vi "模拟器自动控制程序（轨迹跟踪）.vi"() -> ()   [LabVIEW 2012]
uses:
  <vilib>/Utility/error.llb/DialogType.ctl
  <vilib>/Platform/TimedLoop/XDataNode/timing_clust.ctl
  <vilib>/Platform/TimedLoop/XDataNode/nitl_modes.ctl
  <vilib>/Platform/TimedLoop/XDataNode/wakeup.ctl
  <vilib>/Instr/_visa.llb/VISA Configure Serial Port (Instr).vi
  <vilib>/DAQmx/create/channels.llb/DAQmx Create Channel (DO-Digital Output).vi
  <vilib>/Analysis/Matrix/Numeric/Conversions/Array To Matrix - RA2.vi
  <vilib>/Utility/file.llb/Write To Spreadsheet File (DBL).vi
  <vilib>/Platform/TimedLoop/XDataNode/XDataNode.xnode
  <vilib>/Platform/TimedLoop/XDataNode/XDNodeRunTimeDep.lvlib
  <vilib>/Analysis/Matrix/NI_Matrix.lvlib
  <vilib>/vision/NI_Vision_Development_Module.lvlib
  <vilib>/Analysis/NI_AALBase.lvlib
panel:
  out "Truster4":bool
  out "Truster 8":bool
  out "Truster  3":bool
  out "Truster 7":bool
  out "Truster 5":bool
  out "Truster  2":bool
  out "Truster 6":bool
  out "Truster1":bool
  out "定位点信息":T1(array[cluster]) {"Aspect Ratio" format="%.2f"; "Orientation" format="%.2f"; "Area" format="%.2f"; "Object Center"."Y" format="%.2f"; "Object Center"."X" format="%.2f"}
  out "alpha":dbl
  out "计时参数":dbl
  in  "卫星模拟器":enum32{"初始化", "运行监测"}(tab)
  out "读取缓冲区":string
  out "电流校正模式":bool
  out "软件使能":bool caption="软件使能(启动/停止)"
  out "电流校正中":bool caption="电流校正完成"
  out "E2PROM初始化结果":bool
  out "E2初始化完成":bool
  out "CRC校验和错误":bool
  out "串口通信错误":bool caption="串口通信故障"
  out "发送指令":string
  out "控制命令":string
  out "电机已启动":bool
  in  "采样率":i64=10
  in  "限制转速":dbl=500.0
  in  "ID号":u8=255 step=1 format="%#.0f"
  in  "最高转速":dbl=500.0
  in  "PWM周期":dbl=1599.0
  in  "最大力矩":dbl=2047.0
  in  "stop bits (10: 1 bit)":u16(ring)=10 caption="停止位" items=["1.0"=10, "1.5"=15, "2.0"=20]
  out "串口状态":bool
  in  "端口选择":refnum<visa-resource-name>="COM1"
  in  "波特率":u16(ring)=10 items=["   300", "   600", "   1200", "   2400", "   4800   ", "   9600", "   19200", "   38400", "   43000", "   56000", "   57600", "   115200"]
  in  "校验":enum16{"None", "Odd", "Even"}(ring)=enum."Even"
  in  "数据位":u16=8
  in  "打开":bool caption="stop"
  out "轨控信号":dbl
  in  "姿轨控开始":bool
  out "转速模式":bool
  out "转矩模式":bool
  out "故障":bool
  out "启停状态":bool
  in  "存储波形":bool
  in  "显示波形 停止显示":bool
  in  "开始记录":bool
  out "动量轮转矩":dbl format="%#_6f"
  out "动量轮转速":dbl format="%#_4f"
  out "X速率(cm/s)":dbl
  out "Y速率(cm/s)":dbl
  out "Y偏移量 (cm)":dbl
  out "X偏移量 (cm)":dbl
  out "相对偏角(deg)":dbl
  out "角速度(deg/s)":dbl
  out "设备ID":u8=255
  in  "模式选择":u16(ring)=1 items=["电流校正模式", "转矩模式", "转速模式", "开环测试模式"]
  in  "模式选择":bool
  in  "写指令字":dbl
  in  "清除故障":bool
  in  "停止电机":bool
  in  "启动电机":bool
  out "波形图":cluster{"转矩反馈":dbl, "转速反馈":dbl}(graph)
  in  "退出程序":bool caption="停止电机 2"
  in  "Floating":bool
  in  "缩放比例 (像素/cm)":dbl=4.099468
  in  "X中心校正":dbl
  in  "Y中心校正":dbl
  out "指令Y":dbl
  out "指令X":dbl
  out "指令角度":dbl
  out "alpha (deg)":dbl
  out "x >= y?":bool
  out "数值":dbl
  out "输出数组 6":dbl[](array[numeric])
  out "输出数组 7":dbl[](array[numeric])
  out "输出数组 10":dbl[](array[numeric])
  out "无符号字节数组 2":u8[](array[numeric])
  # "状态"
  # "设置"
  # "控制信号"
  # "参数确定"
  # "状态显示"
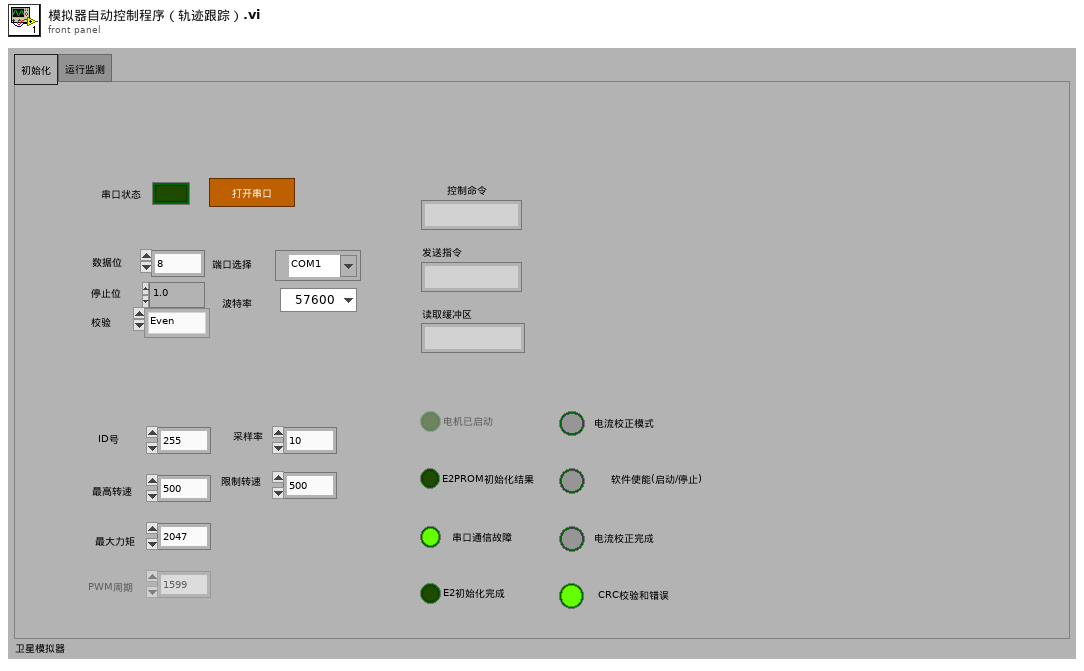
[diagram p1: front panel]
types:
  T1 = cluster{"Object Center":cluster{"X":sgl, "Y":sgl}, "Bounding Box":cluster{"X Left":i32, "Y Top":i32, "X Right":i32, "Y Bottom":i32}, "Area":sgl, "Orientation":sgl, "Aspect Ratio":sgl, "Nb Holes":i32}[]
  T2 = typedef "XDNodeRunTimeDep.lvlib/timing_clust.ctl" = cluster{"Expected End [f-1]":u64, "Actual End [f-1]":u64, "Finished Late? [f-1]":bool, "Expected End [i-1]":u64, "Actual End [i-1]":u64, "Finished Late? [i-1]":bool, "Expected Start [i]":u64, "Actual Start [i]":u64, "Expected Start [f]":u64, "Actual Start [f]":u64, "Source Name":string, "Structure Name":string, "Period":i64, "Deadline":i64, "Offset":i64, "Start":i64, "Priority":i32, "Timeout":i32, "Mode":T3, "Wakeup Reason":T4, "Error":errorcluster, "Source Type":string, "Secondary Source Type":string, "Global End Time":u64, "Global Start Time":u64, "Frame Duration":u64, "Iteration Duration":u64, "Assigned CPU":i32, "I/O Scan Engine Mode":u32}
  T3 = typedef "XDNodeRunTimeDep.lvlib/nitl_modes.ctl" = enum32{"No Change", "Process missed periods, maintain original phase", "Discard missed periods, maintain original phase", "Process missed periods, ignore original phase", "Discard missed periods, ignore original phase"}
  T4 = typedef "XDNodeRunTimeDep.lvlib/wakeup.ctl" = enum32{"Normal", "Aborted", "Asynchronous wakeup", "Timing source error", "Timed loop error", "Timeout"}
  T5 = cluster{"Objects":u16, "Threshold":i32, "Reject Border":bool, "Fill Holes":bool, "Min Object Size":bool, "Min Size":i32, "Max Object Size":bool, "Max Size":i32, "Show Search Area":bool, "Show Center":bool, "Show Bounding Box":bool}
  T6 = typedef "DialogType.ctl" = u16
  T7 = typedef "NI_Matrix.lvlib/RealMatrix.ctl" = dbl[][]
  T8 = typedef "IMAQ Image.ctl" = refnum<image>
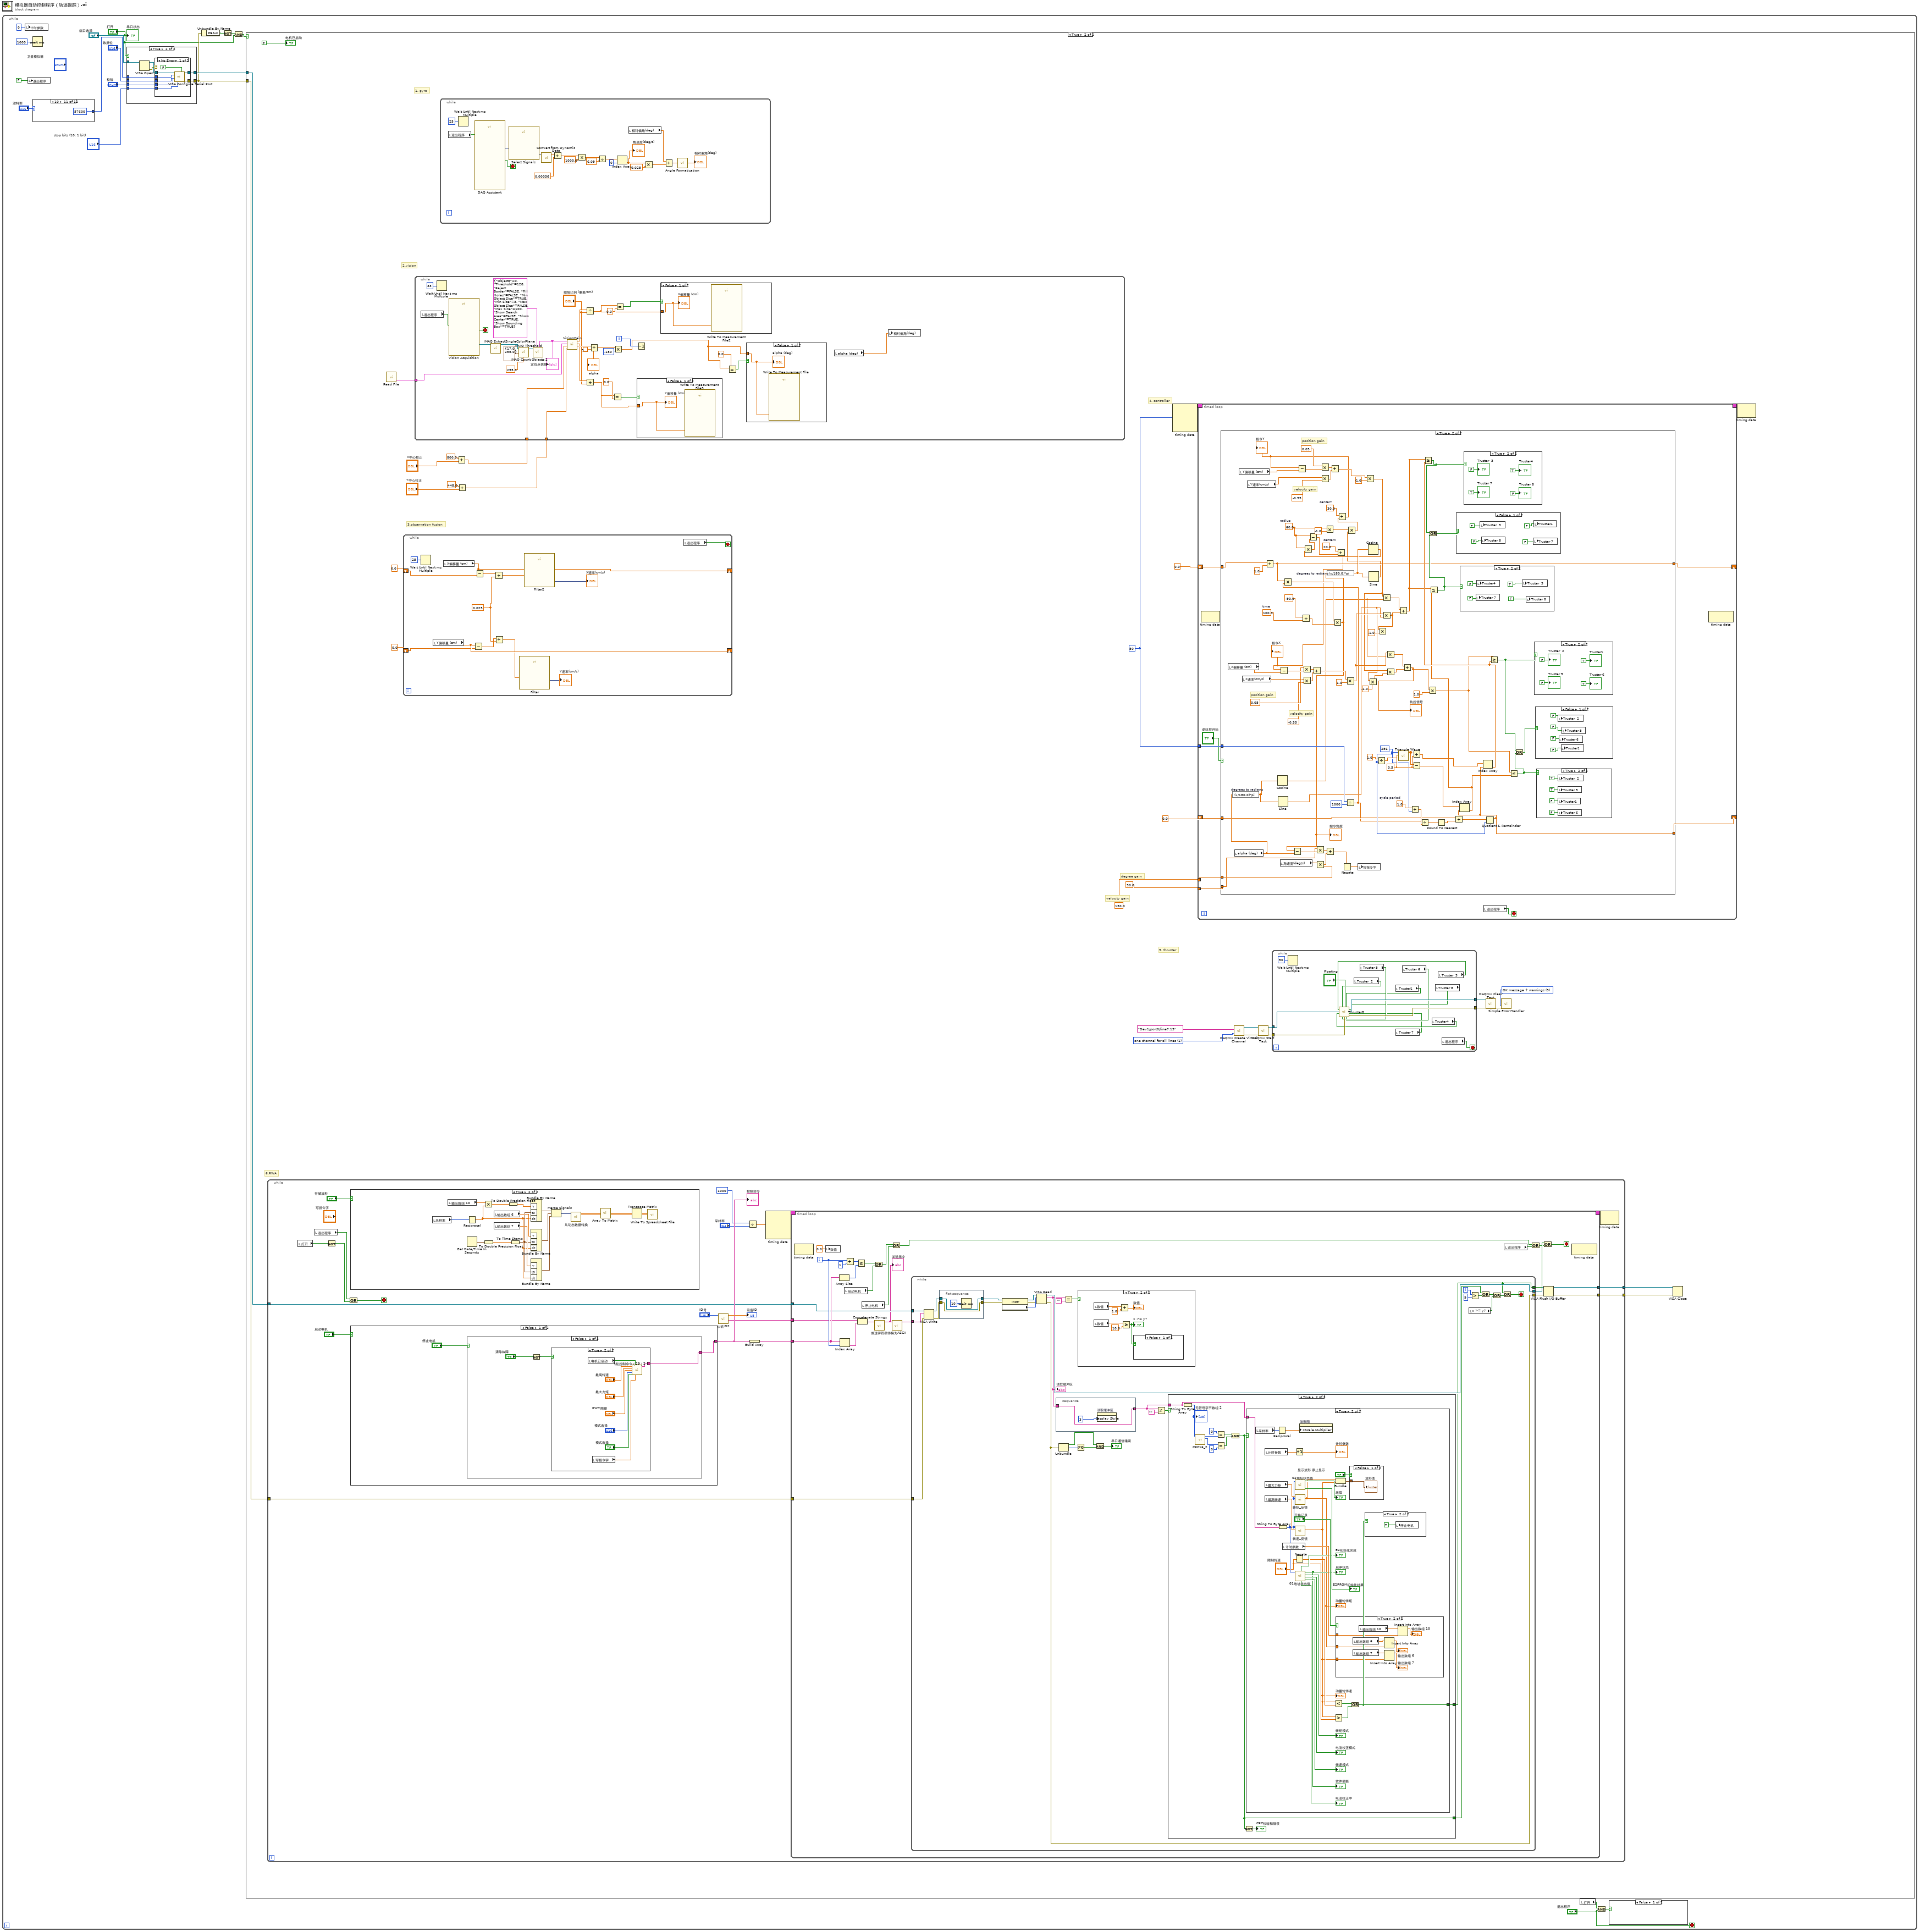
[diagram p0: block diagram]
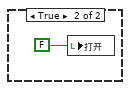
[diagram p2: hidden frame]
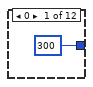
[diagram p5: hidden frame]
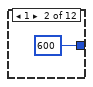
[diagram p6: hidden frame]
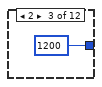
[diagram p7: hidden frame]
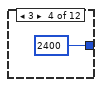
[diagram p8: hidden frame]
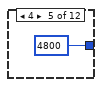
[diagram p9: hidden frame]
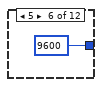
[diagram p10: hidden frame]
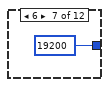
[diagram p11: hidden frame]
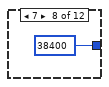
[diagram p12: hidden frame]
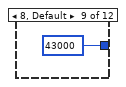
[diagram p13: hidden frame]
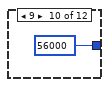
[diagram p14: hidden frame]
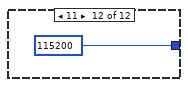
[diagram p15: hidden frame]
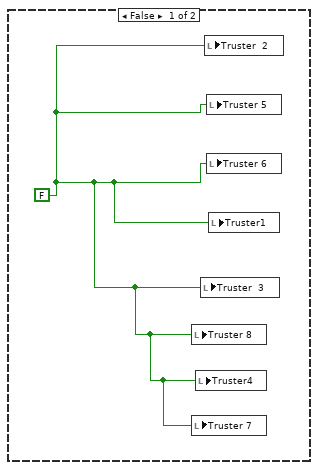
[diagram p17: hidden frame]
diagram:
  n1 = while {
    stop <- "退出程序" stop-if-true
    n2 = local write "计时参数"(0) -> ()
    n3 = local write "退出程序"(FALSE ("退出程序")) -> ()
    n4 = Wait (ms)(milliseconds to wait=u32 1000 ("等待时间（毫秒）")) -> ()  [unwired: 1 out]
    n5 = case shown="10" "波特率" {
      tunnel: [300 600 1200 2400 4800 9600 19200 38400 43000 56000 57600 115200] -> w17
      frame 0 {
      }
      frame 1 {
      }
      frame 2 {
      }
      frame 3 {
      }
      frame 4 {
      }
      frame 5 {
      }
      frame 6 {
      }
      frame 7 {
      }
      frame 8, Default {
      }
      frame 9 {
      }
      frame 10 {
      }
      frame 11 {
      }
    }
    n6 = case shown="True" "打开" {
      tunnel: w17 -> [_ w28]
      tunnel: "数据位" -> [_ w27]
      tunnel: "校验" -> [_ w26]
      tunnel: "端口选择" -> [_ w25]
      tunnel: [_ w22] -> w7
      tunnel: [_ w21] -> w6
      tunnel: "stop bits (10: 1 bit)" -> [_ w20]
      frame False {
      }
      frame True {
        n7 = VISA Open(VISA resource name=w25) -> (VISA resource name=w24:refnum<visa-resource-name>, error out=w23:errorcluster)  [unwired: 1 in, 3 out]
        n8 = case shown="No Error" w23 {
          tunnel: w28 -> [w36 _]
          tunnel: w27 -> [w35 _]
          tunnel: w26 -> [w34 _]
          tunnel: w24 -> [w33 _]
          tunnel: [w32 _] -> w22
          tunnel: [w31 _] -> w21
          tunnel: w20 -> [w30 _]
          frame No Error {
            n9 = call-poly "VISA Configure Serial Port"("VISA resource name"=w33, "Enable Termination\nChar (T)"=FALSE ("Enable Termination\nChar (T)"), "baud rate (9600)"=w36, "data bits (8)"=w35, "parity (0:none)"=w34, "stop bits (10: 1 bit)"=w30) -> ("VISA resource name out"=w32:refnum<visa-resource-name>, "error out"=w31:errorcluster)  [unwired: 2 in, 6 out]
          }
          frame Error {
          }
        }
      }
    }
    n10 = Unbundle By Name(w6) -> ("status"=w12:bool)
    n11 = Not(x=w12) -> (.not. x?=w11:bool)
    n12 = And(x=w11, y="打开") -> (x .and. y?=w8:bool)
    n13 = case shown="True" w8 {
      tunnel: w7 -> [_ w76]
      tunnel: w6 -> [_ w75]
      frame False {
      }
      frame True {
        w56 = 1 items=["one channel for each line", "one channel for all lines"] ("line grouping")
        w58 = T6 3 items=["no dialog", "OK message", "continue or stop message", "OK message + warnings", "continue/stop + warnings"] ("type of dialog (OK msg:1)")
        w52 = 50
        # "5. thruster"
        # "6.RWA"
        # "4. controller"
        # "3.observation fusion"
        # "2.vision"
        # "1. gyro"
        # "velocity gain"
        # "degree gain"
        n14 = while {
          tunnel: [w297] -> w78
          tunnel: [w296] -> w77
          tunnel: w76 -> [w295]
          tunnel: w75 -> [w294]
          stop <- w290 stop-if-true
          n15 = local read "打开"() -> (w293:bool)
          n16 = local read "退出程序"() -> (w292:bool)
          n17 = Not(x=w293) -> (.not. x?=w291:bool)
          n18 = Or(x=w292, y=w291) -> (x .or. y?=w290:bool)
          n19 = case shown="True" "存储波形" {
            frame False {
            }
            frame True {
              n20 = local read "采样率"() -> (w322:i64)
              n21 = local read "输出数组 10"() -> (w315:dbl[])
              n22 = Reciprocal(x=w322) -> (1/x=w317:dbl)
              n23 = Get Date/Time In Seconds() -> (seconds since 1Jan1904=w326:timestamp)
              n24 = Multiply(x=w315, y=w317) -> (x*y=w316:dbl[])
              n25 = To Double Precision Float(number=w326) -> (double precision float=w325:dbl)
              n26 = local read "输出数组 6"() -> (w324:dbl[])
              n27 = local read "输出数组 7"() -> (w323:dbl[])
              n28 = To Double Precision Float(number=w316) -> (double precision float=w314:dbl[])
              n29 = To Time Stamp(1:w325) -> (0:w318:timestamp)
              n30 = Bundle By Name("Y"=w314, "t0"=w318, "dt"=w317) -> (w319:waveform(dbl))  [unwired: 1 out]
              n31 = Bundle By Name("Y"=w324, "t0"=w318, "dt"=w317) -> (w320:waveform(dbl))  [unwired: 1 out]
              n32 = Bundle By Name("Y"=w323, "t0"=w318, "dt"=w317) -> (w321:waveform(dbl))  [unwired: 1 out]
              n33 = Merge Signals(w319, w320, w321) -> (w313:dynamicdata)
              n34 = call "从动态数据转换"("Dynamic Data Type"=w313) -> ("Array"=w312:dbl[][])  [unwired: 3 in]
              n35 = call-poly <vilib>:"Array To Matrix.vi"("Real 2D Array"=w312) -> ("Real Matrix"=w311:T7)
              n36 = Transpose Matrix(1:w311) -> (0:w310:T7)
              n37 = call-poly <vilib>:"Write To Spreadsheet File.vi"("2D data"=w310) -> ()  [unwired: 7 in, 1 out]
            }
          }
          n38 = case shown="False" "启动电机" {
            tunnel: [w453 w480] -> w306
            frame False {
              n39 = case shown="False" "停止电机" {
                tunnel: [w454 w473] -> w453
                frame False {
                  n40 = Not(x="清除故障") -> (.not. x?=w455:bool)
                  n41 = case shown="True" w455 {
                    tunnel: [w457 w466] -> w454
                    frame False {
                      n42 = call <vilib>:"Space Constant.vi"() -> ("String"=w461:string)
                      n43 = Concatenate Strings(w461, "05" ("字符串"), w461, "23" ("字符串"), w461, "01" ("字符串")) -> (w457:string)
                    }
                    frame True {
                      n44 = local read "电机已启动"() -> (w463:bool)
                      n45 = local read "写指令字"() -> (w462:dbl)
                      n46 = call "飞轮控制命令（29）2.vi"("最高转速"="最高转速", "电机启动控制指令"=w463, "力矩最大值"="最大力矩", "pwmperiod"="PWM周期", "模式选择 3"="模式选择", "模式选择 4"="模式选择", "写指令字"=w462) -> ("字符串"=w466:string)  [unwired: 8 in]
                    }
                  }
                }
                frame True {
                  n47 = local write "启动电机"(FALSE ("停止电机")) -> ()
                  n48 = local write "停止电机"(FALSE ("停止电机")) -> ()
                  n49 = local write "电机已启动"(FALSE) -> ()
                  n50 = call <vilib>:"Space Constant.vi"() -> ("String"=w477:string)
                  n51 = Concatenate Strings(w477, "05" ("字符串"), w477, "22" ("字符串"), w477, "00" ("字符串")) -> (w473:string)
                }
              }
            }
            frame True {
              n52 = local write "启动电机"(FALSE) -> ()
              n53 = local write "电机已启动"(TRUE) -> ()
              n54 = call <vilib>:"Space Constant.vi"() -> ("String"=w484:string)
              n55 = Concatenate Strings(w484, "05" ("字符串"), w484, "22" ("字符串"), w484, "01" ("字符串")) -> (w480:string)
            }
          }
          "控制命令" <- w306
          n56 = call "从机ID2.vi"("ID号"="ID号") -> ("字符串"=w298:string, "设备ID"=→"设备ID":dbl)  [unwired: 9 in]
          n57 = Divide(x=i64 1000 ("Period"), y="采样率") -> (x/y=w302:dbl)
          n58 = Build Array(w306) -> (w303:string[])
          n59 = node-c288(w302) -> (w305:T2)  [unwired: 3 in]
          n60 = timed-loop {
            timing: w305 -> [_]
            timing-out: [_] -> w304
            tunnel: w303 -> [w347]
            tunnel: w298 -> [w343]
            tunnel: [w340] -> w297
            tunnel: [w339] -> w296
            tunnel: w295 -> [w338]
            tunnel: w294 -> [w337]
            i -> [w346]
            stop <- w327 stop-if-true
            n61 = node-c288() -> ()  [unwired: 1 in, 1 out]
            n62 = local write "数值"(0.0 ("y")) -> ()
            n63 = Array Size(array=w347) -> (size(s)=w351:i32)
            n64 = Index Array(array=w347, index=w346) -> (element=w350:string)
            n65 = local read "启动电机"() -> (w334:bool)
            n66 = Add(x=w346, y=1) -> (x+y=w352:i32)
            n67 = Greater Or Equal?(x=w352, y=w351) -> (x >= y?=w335:bool)
            n68 = Concatenate Strings(w343, w350) -> (w349:string)
            n69 = local read "停止电机"() -> (w333:bool)
            n70 = Or(x=w335, y=w334) -> (x .or. y?=w332:bool)
            n71 = call "发送字符串.vi"("字符串"=w349) -> ("连接的字符串 2"=w336:string)  [unwired: 10 in]
            "发送指令" <- w336
            n72 = Or(x=w332, y=w333) -> (x .or. y?=w330:bool)
            n73 = call "转换为ASCII.vi"("字符串"=w336) -> ("字符串 2"=w348:string)  [unwired: 10 in]
            n74 = while {
              tunnel: [w380] -> w341
              tunnel: [w369] -> w342
              tunnel: w348 -> [w374]
              tunnel: w338 -> [w355]
              tunnel: w337 -> [w354]
              tunnel: [w353] -> w329
              i -> [w379]
              stop <- w362 stop-if-true
              n75 = VISA Write(VISA resource name=w355, write buffer=w374, error in (no error)=w354) -> (VISA resource name out=w360:refnum<visa-resource-name>, error out=w357:errorcluster)  [unwired: 1 out]
              n76 = flat-sequence {
                tunnel: w360 -> [w386]
                tunnel: [w386] -> w359
                tunnel: [w385] -> w358
                tunnel: w357 -> [w385]
                frame #0 {
                  n77 = Wait (ms)(milliseconds to wait=i64 10 ("Period")) -> ()  [unwired: 1 out]
                }
              }
              n78 = property class="Instr"(reference=w359, error in=w358) -> (reference out=w382:refnum<visa-resource-name>, error out=w381:errorcluster, "Serial Settings:Number of Bytes at Serial Port"=w383:u32)
              n79 = VISA Read(VISA resource name=w382, byte count=w383, error in (no error)=w381) -> (VISA resource name out=w380:refnum<visa-resource-name>, read buffer=w373:string, error out=w369:errorcluster)  [unwired: 1 out]
              "读取缓冲区" <- w373
              n80 = stacked-sequence {
                tunnel: [w437] -> w372
                tunnel: w373 -> [w437]
                frame #0 {
                  n81 = property on="读取缓冲区" class="Str"("Display Style"=u32 3 ("显示样式")) -> ()  [unwired: 2 in, 2 out]
                }
              }
              n82 = Unbundle(w369) -> ("status"=w366:bool, "code"=w368:i32)  [unwired: 1 out]
              n83 = Equal?(x=w373, y="") -> (x = y?=w376:bool)
              n84 = Not Equal To 0?(x=w368) -> (x != 0?=w367:bool)
              n85 = case shown="True" w376 {
                frame False {
                  n86 = local write "数值"(0.0 ("数值")) -> ()
                }
                frame True {
                  n87 = local read "数值"() -> (w439:dbl)
                  n88 = local read "数值"() -> (w444:dbl)
                  n89 = Add(x=w439, y=1.0) -> (x+y=→"数值":dbl)
                  n90 = Greater Or Equal?(x=w444, y=10.0) -> (x >= y?=w442:bool)
                  "x >= y?" <- w442
                  n91 = case shown="False" w442 {
                    frame False {
                    }
                    frame True {
                      n92 = local write "打开"(FALSE) -> ()
                    }
                  }
                }
              }
              n93 = And(x=w366, y=w367) -> (x .and. y?=→"串口通信错误":bool)
              n94 = Not Equal?(x=w372, y="") -> (x != y?=w361:bool)
              n95 = case shown="True" w361 {
                tunnel: w372 -> [_ w397]
                tunnel: [_ w391] -> w370
                tunnel: [_ w392] -> w353
                frame False {
                }
                frame True {
                  n96 = String To Byte Array(string=w397) -> (unsigned byte array=w387:u8[])
                  "无符号字节数组 2" <- w387
                  n97 = call "CRC16_2.vi"("buf"=w387) -> ("CRCHi"=w388:u8, "CRCLo"=w389:u8)  [unwired: 9 in]
                  n98 = Equal?(x=u8 0, y=w389) -> (x = y?=w393:bool)
                  n99 = Equal?(x=w388, y=u8 0) -> (x = y?=w394:bool)
                  n100 = And(x=w393, y=w394) -> (x .and. y?=w391:bool)
                  n101 = Not(x=w391) -> (.not. x?=→"CRC校验和错误":bool)
                  n102 = case shown="True" w391 {
                    tunnel: w397 -> [_ w424]
                    tunnel: [_ w398] -> w392
                    frame False {
                    }
                    frame True {
                      n103 = local read "采样率"() -> (w422:i64)
                      n104 = local read "计时参数"() -> (w419:dbl)
                      n105 = local read "最大力矩"() -> (w407:dbl)
                      n106 = local read "最高转速"() -> (w405:dbl)
                      n107 = Reciprocal(x=w422) -> (1/x=w421:dbl)
                      n108 = String To Byte Array(string=w424) -> (unsigned byte array=w404:u8[])
                      n109 = local read "计时参数"() -> (w416:dbl)
                      n110 = Increment(x=w419) -> (x+1=→"计时参数":dbl)
                      n111 = Negate(x="限制转速") -> (-x=w403:dbl)
                      n112 = call "02地址状态值.vi"("unsigned byte array"=w404) -> ("E2初始化失败"=→"E2PROM初始化结果":bool, "故障"=→"故障":bool)  [unwired: 9 in]
                      n113 = call "转矩_反馈.vi"("unsigned byte array"=w404, "最大转矩"=w407) -> ("转矩反馈"=w406:dbl)  [unwired: 9 in]
                      "动量轮转矩" <- w406
                      n114 = call "转速_反馈.vi"("最高转速"=w405, "unsigned byte array"=w404) -> ("转速反馈"=w402:dbl)  [unwired: 9 in]
                      "动量轮转速" <- w402
                      n115 = call "01地址状态值.vi"("unsigned byte array"=w404) -> ("E2初始化完成"=→"E2初始化完成":bool, "电流校正完成"=→"电流校正中":bool, "启停状态"=→"软件使能" →"启停状态":bool, "转矩模式"=→"转矩模式":bool, "电流校正"=→"电流校正模式":bool, "转速模式"=→"转速模式":bool)  [unwired: 4 in]
                      n116 = property on="波形图" class="WFChart (strict)"("XScale.Multiplier"=w421) -> ()  [unwired: 2 in, 2 out]
                      n117 = Less?(x=w402, y=w403) -> (x < y?=w399:bool)
                      n118 = Greater?(x=w402, y="限制转速") -> (0:w400:bool)
                      n119 = Bundle("转矩反馈"=w406, "转速反馈"=w402) -> (w423:cluster{"转矩反馈":dbl, "转速反馈":dbl})  [unwired: 1 out]
                      n120 = case shown="True" "开始记录" {
                        tunnel: w406 -> [_ w428]
                        tunnel: w402 -> [_ w427]
                        tunnel: w416 -> [_ w426]
                        frame False {
                        }
                        frame True {
                          n121 = local read "输出数组 6"() -> (w433:dbl[])
                          n122 = local read "输出数组 7"() -> (w431:dbl[])
                          n123 = local read "输出数组 10"() -> (w429:dbl[])
                          n124 = Insert Into Array(array=w433, new element=w428) -> (→"输出数组 6":dbl[])  [unwired: 1 in]
                          n125 = Insert Into Array(array=w431, new element=w427) -> (→"输出数组 7":dbl[])  [unwired: 1 in]
                          n126 = Insert Into Array(array=w429, new element=w426) -> (→"输出数组 10":dbl[])  [unwired: 1 in]
                        }
                      }
                      n127 = case shown="False" "显示波形 停止显示" {
                        tunnel: w423 -> [w435 _]
                        frame False {
                          "波形图" <- w435
                        }
                        frame True {
                        }
                      }
                      n128 = Or(x=w399, y=w400) -> (x .or. y?=w398:bool)
                      n129 = case shown="True" w398 {
                        frame False {
                        }
                        frame True {
                          n130 = local write "停止电机"(TRUE ("停止电机")) -> ()
                        }
                      }
                    }
                  }
                }
              }
              n131 = local read "x >= y?"() -> (w364:bool)
              n132 = Greater?(x=w379, y=9) -> (0:w356:bool)
              n133 = Or(x=w370, y=w356) -> (x .or. y?=w375:bool)
              n134 = Or(x=w375, y=w364) -> (x .or. y?=w363:bool)
              n135 = Or(x=w353, y=w363) -> (x .or. y?=w362:bool)
            }
            n136 = local read "退出程序"() -> (w331:bool)
            n137 = Or(x=w330, y=w331) -> (x .or. y?=w328:bool)
            n138 = Or(x=w329, y=w328) -> (x .or. y?=w327:bool)
            n139 = VISA Flush I/O Buffer(VISA resource name=w341, error in (no error)=w342) -> (VISA resource name out=w340:refnum<visa-resource-name>, error out=w339:errorcluster)  [unwired: 1 out]
            n140 = node-c288() -> ()  [unwired: 1 in, 1 out]
          }
          n141 = node-c288(w304) -> ()  [unwired: 1 out]
        }
        n142 = call "Read File.vi"() -> ("Objects"=w73:T1)  [unwired: 1 in, 1 out]
        n143 = while {
          shift-right: [w283] -> _
          shift-left: 0.0 ("X偏移量 (cm)") -> [w282]
          shift-right: [w280] -> _
          shift-left: 0.0 ("Y偏移量 (cm)") -> [w279]
          stop <- w288 stop-if-true
          w281 = 0.025 ("y")
          n144 = Wait Until Next ms Multiple(millisecond multiple=u32 25) -> ()  [unwired: 1 out]
          n145 = local read "Y偏移量 (cm)"() -> (w280:dbl)
          n146 = local read "X偏移量 (cm)"() -> (w283:dbl)
          n147 = Subtract(x=w280, y=w279) -> (x-y=w285:dbl)
          n148 = Subtract(x=w283, y=w282) -> (x-y=w286:dbl)
          n149 = Divide(x=w286, y=w281) -> (x/y=w277:dbl)
          n150 = Divide(x=w285, y=w281) -> (x/y=w278:dbl)
          n151 = call "Filter"("Signal"=w278) -> ("Filtered Signal"=→"Y速率(cm/s)":dynamicdata)  [unwired: 9 in, 1 out]
          n152 = call "Filter2"("Signal"=w277) -> ("Filtered Signal"=→"X速率(cm/s)":dynamicdata)  [unwired: 9 in, 1 out]
          n153 = local read "退出程序"() -> (w288:bool)
        }
        n154 = while {
          stop <- w276 stop-if-true
          n155 = local read "退出程序"() -> (w263:bool)
          n156 = Wait Until Next ms Multiple(millisecond multiple=u32 25 ("y")) -> ()  [unwired: 1 out]
          n157 = call "DAQ Assistant"("stop (F)"=w263) -> ("data"=w261:dynamicdata, "stopped"=w276:bool)  [unwired: 15 in, 2 out]
          n158 = call "Select Signals"("Signals"=w261) -> ("Signal Out"=w262:dynamicdata)  [unwired: 9 in, 1 out]
          n159 = call "Convert from Dynamic Data"("Dynamic Data Type"=w262) -> ("Array"=w267:dbl[])  [unwired: 3 in]
          n160 = Add(x=w267, y=0.00036) -> (x+y=w265:dbl[])
          n161 = Multiply(x=w265, y=1000.0) -> (x*y=w275:dbl[])
          n162 = Divide(x=w275, y=6.09) -> (x/y=w269:dbl[])
          n163 = Index Array(array=w269, index=0) -> (element=w259:dbl)
          "角速度(deg/s)" <- w259
          n164 = local read "相对偏角(deg)"() -> (w264:dbl)
          n165 = Multiply(x=w259, y=0.025) -> (x*y=w270:dbl)
          n166 = Add(x=w264, y=w270) -> (x+y=w260:dbl)
          n167 = call "Angle Formatization.vi"("Alpha"=w260) -> ("Alpha Formatized"=→"相对偏角(deg)":dbl)
        }
        n168 = Add(x=800.0 ("c_x"), y="X中心校正") -> (x+y=w70:dbl)
        n169 = Add(x=448.0 ("c_y"), y="Y中心校正") -> (x+y=w67:dbl)
        n170 = while {
          tunnel: w73 -> [w229]
          tunnel: w67 -> [w223]
          tunnel: w70 -> [w222]
          i -> [w225]
          stop <- w239 stop-if-true
          n171 = local read "退出程序"() -> (w231:bool)
          n172 = Wait Until Next ms Multiple(millisecond multiple=u32 33 ("y")) -> ()  [unwired: 1 out]
          n173 = call "Vision Acquisition"("Stop (F)"=w231) -> ("Image Out"=w235:T8, "Stopped"=w239:bool)  [unwired: 24 in, 1 out]
          n174 = call "IMAQ ExtractSingleColorPlane"("Image Src"=w235) -> ("Image Dst Out"=w220:T8)  [unwired: 9 in, 1 out]
          n175 = call "IMAQ Threshold"("Replace Value"=sgl 255.0 ("replace value"), "Range"=cluster{"lower value":sgl, "upper value":sgl} {"lower value"=17.0, "upper value"=255.0} ("threshold"), "Image Src"=w220) -> ("Image Dst Out"=w236:T8)  [unwired: 7 in, 1 out]
          n176 = call "IMAQ Count Objects 2"("Settings"=T5 {"Objects"=0, "Threshold"=128, "Reject Border"=FALSE, "Fill Holes"=FALSE, "Min Object Size"=TRUE, "Min Size"=3, "Max Object Size"=FALSE, "Max Size"=100, "Show Search Area"=FALSE, "Show Center"=TRUE, "Show Bounding Box"=TRUE}, "Image"=w236) -> ("Objects"=w230:T1)  [unwired: 5 in, 4 out]
          "定位点信息" <- w230
          n177 = call "VisionMain.vi"("Y Center"=w223, "X Center"=w222, "Original Plots"=w229, "Plots Captured"=w230) -> ("alpha"=w228:dbl, "dy"=w227:dbl, "dx"=w226:dbl)  [unwired: 5 in]
          "alpha" <- w228
          n178 = Divide(x=w226, y="缩放比例 (像素/cm)") -> (x/y=w214:dbl)
          n179 = Divide(x=w227, y="缩放比例 (像素/cm)") -> (x/y=w211:dbl)
          n180 = Divide(x=w228, y=3.141592653589793) -> (x/y=w233:dbl)
          n181 = Equal?(x=w211, y=0.0) -> (x = y?=w212:bool)
          n182 = Multiply(x=w233, y=-180) -> (x*y=w217:dbl)
          n183 = Equal?(x=w214, y=0.0) -> (x = y?=w215:bool)
          n184 = Decrement(x=w225) -> ()  [unwired: 1 out]
          n185 = case shown="False" w212 {
            tunnel: w211 -> [w240 _]
            frame False {
              n186 = call "Write To Measurement File3"("Signals"=w240) -> ()  [unwired: 16 in, 3 out]
              "Y偏移量 (cm)" <- w240
            }
            frame True {
            }
          }
          n187 = case shown="False" w215 {
            tunnel: w214 -> [w241 _]
            frame False {
              n188 = call "Write To Measurement File2"("Signals"=w241) -> ()  [unwired: 16 in, 3 out]
              "X偏移量 (cm)" <- w241
            }
            frame True {
            }
          }
          n189 = Equal?(x=w217, y=0.0) -> (x = y?=w218:bool)
          n190 = case shown="False" w218 {
            tunnel: w217 -> [w242 _]
            frame False {
              n191 = call "Write To Measurement File"("Signals"=w242) -> ()  [unwired: 16 in, 3 out]
              "alpha (deg)" <- w242
            }
            frame True {
            }
          }
          n192 = local read "alpha (deg)"() -> (w210:dbl)
          n193 = local write "相对偏角(deg)"(w210) -> ()
        }
        n194 = node-c288(w52) -> (w54:T2)  [unwired: 3 in]
        n195 = timed-loop {
          tunnel: 30.0 ("degree gain") -> [w88]
          tunnel: 130.0 ("angular velocity gain") -> [w87]
          shift-right: [w86] -> _
          shift-left: 0.0 -> [w85]
          tunnel: w52 -> [w84]
          timing: w54 -> [_]
          timing-out: [_] -> w53
          shift-right: [w81] -> _
          shift-left: 0.0 -> [w80]
          stop <- w83 stop-if-true
          n196 = node-c288() -> ()  [unwired: 1 in, 1 out]
          n197 = case shown="True" "姿轨控开始" {
            tunnel: w88 -> [_ w176]
            tunnel: w87 -> [_ w175]
            tunnel: [_ w147] -> w86
            tunnel: w85 -> [_ w146]
            tunnel: w84 -> [_ w145]
            tunnel: [_ w110] -> w81
            tunnel: w80 -> [_ w127]
            frame False {
              w89 = FALSE ("Truster 6")
              n198 = local write "Truster 8"(w89) -> ()
              n199 = local write "Truster 7"(w89) -> ()
              n200 = local write "Truster4"(w89) -> ()
              n201 = local write "Truster  3"(w89) -> ()
              n202 = local write "Truster  2"(w89) -> ()
              n203 = local write "Truster 5"(w89) -> ()
              n204 = local write "Truster 6"(w89) -> ()
              n205 = local write "Truster1"(w89) -> ()
            }
            frame True {
              w103 = 20.0  # centerX
              w107 = 30.0  # centerY
              w109 = 60.0  # radius
              w125 = 100.0  # time
              w151 = 256 ("samples")
              w158 = 1.0  # cycle period
              w162 = 0.5 ("amplitude")
              # "position gain"
              # "velocity gain"
              # "velocity gain"
              # "position gain"
              n206 = local read "X偏移量 (cm)"() -> (w169:dbl)
              n207 = local read "alpha (deg)"() -> (w90:dbl)
              n208 = expression code="(x/180.0)*pi" "degrees to radians"(w90) -> (w93:dbl)
              n209 = local read "Y偏移量 (cm)"() -> (w138:dbl)
              n210 = local read "X速率(cm/s)"() -> (w167:dbl)
              n211 = local read "Y速率(cm/s)"() -> (w136:dbl)
              n212 = Add(x=w127, y=1.0) -> (x+y=w110:dbl)
              n213 = Cosine(x=w93) -> (cos(x)=w91:dbl)
              n214 = Sine(x=w93) -> (sin(x)=w92:dbl)
              n215 = local read "角速度(deg/s)"() -> (w171:dbl)
              n216 = Divide(x=-90.0 ("time"), y=w125) -> (x/y=w123:dbl)
              n217 = Multiply(x=w167, y=-0.55) -> (x*y=w165:dbl)
              n218 = Multiply(x=w171, y=w175) -> (x*y=w174:dbl)
              n219 = Multiply(x=w136, y=-0.55) -> (x*y=w140:dbl)
              n220 = Multiply(x=w109, y=-1.0) -> (x*y=w106:dbl)
              n221 = Divide(x=w145, y=u32 1000) -> (x/y=w124:dbl)
              n222 = Multiply(x=w110, y=w124) -> (x*y=w111:dbl)
              n223 = Multiply(x=w111, y=w123) -> (x*y=w94:dbl)
              "指令角度" <- w94
              n224 = Subtract(x=w94, y=w90) -> (x-y=w178:dbl)
              n225 = Multiply(x=w176, y=w178) -> (x*y=w177:dbl)
              n226 = Add(x=w177, y=w174) -> (x+y=w173:dbl)
              n227 = expression code="(x/180.0)*pi" "degrees to radians"(w94) -> (w122:dbl)
              n228 = Negate(x=w173) -> (-x=w172:dbl)
              n229 = local write "写指令字"(w172) -> ()
              n230 = Cosine(x=w122) -> (cos(x)=w113:dbl)
              n231 = Multiply(x=w109, y=w113) -> (x*y=w121:dbl)
              n232 = Subtract(x=w109, y=w121) -> (x-y=w102:dbl)
              n233 = Add(x=w103, y=w102) -> (x+y=w101:dbl)
              "指令X" <- w101
              n234 = Subtract(x=w101, y=w169) -> (x-y=w170:dbl)
              n235 = Multiply(x=0.05 ("degree gain"), y=w170) -> (x*y=w164:dbl)
              n236 = Add(x=w164, y=w165) -> (x+y=w143:dbl)
              n237 = Multiply(x=w143, y=1.0) -> (x*y=w114:dbl)
              n238 = Multiply(x=w92, y=-1.0) -> (x*y=w97:dbl)
              n239 = Sine(x=w122) -> (sin(x)=w96:dbl)
              n240 = Multiply(x=w106, y=w96) -> (x*y=w105:dbl)
              n241 = Add(x=w107, y=w105) -> (x+y=w104:dbl)
              "指令Y" <- w104
              n242 = Subtract(x=w104, y=w138) -> (x-y=w142:dbl)
              n243 = Multiply(x=0.05 ("degree gain"), y=w142) -> (x*y=w139:dbl)
              n244 = Add(x=w139, y=w140) -> (x+y=w129:dbl)
              n245 = Multiply(x=w129, y=-1.0) -> (x*y=w112:dbl)
              n246 = Divide(x=1.0 ("amplitude"), y=w151) -> (x/y=w159:dbl)
              n247 = Multiply(x=w112, y=w91) -> (x*y=w119:dbl)
              n248 = Multiply(x=w114, y=w92) -> (x*y=w118:dbl)
              n249 = Multiply(x=w118, y=-1.0) -> ()  [unwired: 1 out]
              n250 = Multiply(x=w114, y=w91) -> (x*y=w116:dbl)
              n251 = Multiply(x=w112, y=w97) -> (x*y=w115:dbl)
              n252 = call <vilib>:"Triangle Wave.vi"("samples"=w151, "amplitude"=w162, "frequency"=w159) -> ("triangle wave"=w163:dbl[])  [unwired: 2 in, 2 out]
              n253 = Add(x=w119, y=w118) -> (x+y=w117:dbl)
              n254 = Add(x=w116, y=w115) -> (x+y=w100:dbl)
              "轨控信号" <- w100
              n255 = Divide(x=w158, y=w151) -> (x/y=w157:dbl)
              n256 = Add(x=w163, y=w162) -> (x+y=w155:dbl[])
              n257 = Subtract(x=w163, y=w162) -> (x-y=w154:dbl[])
              n258 = Divide(x=w124, y=w157) -> (x/y=w156:dbl)
              n259 = Multiply(x=w100, y=1.0) -> (x*y=w98:dbl)
              n260 = Round To Nearest(number=w156) -> (nearest integer value=w153:dbl)
              n261 = Add(x=w146, y=w153) -> (x+y=w152:dbl)
              n262 = Quotient & Remainder(x=w152, y=w151) -> (x-y*floor(x/y)=w147:dbl)  [unwired: 1 out]
              n263 = Index Array(array=w154, index=w147) -> (element=w134:dbl)
              n264 = Less Or Equal?(x=w117, y=w134) -> (x <= y?=w132:bool)
              n265 = case shown="True" w132 {
                frame False {
                }
                frame True {
                  n266 = local write "Truster 7"(FALSE ("Truster 6")) -> ()
                  n267 = local write "Truster4"(FALSE ("Truster 6")) -> ()
                  n268 = local write "Truster  3"(TRUE ("Truster 6")) -> ()
                  n269 = local write "Truster 8"(TRUE ("Truster 6")) -> ()
                }
              }
              n270 = Index Array(array=w155, index=w147) -> (element=w135:dbl)
              n271 = Greater Or Equal?(x=w117, y=w135) -> (x >= y?=w133:bool)
              n272 = Or(x=w133, y=w132) -> (x .or. y?=w131:bool)
              n273 = case shown="False" w131 {
                frame False {
                  n274 = local write "Truster  3"(FALSE ("Truster 6")) -> ()
                  n275 = local write "Truster 8"(FALSE ("Truster 6")) -> ()
                  n276 = local write "Truster 7"(FALSE ("Truster 6")) -> ()
                  n277 = local write "Truster4"(FALSE ("Truster 6")) -> ()
                }
                frame True {
                }
              }
              n278 = case shown="True" w133 {
                frame False {
                }
                frame True {
                  "Truster4" <- TRUE ("Truster 6")
                  "Truster 8" <- FALSE ("Truster 6")
                  "Truster  3" <- FALSE ("Truster 6")
                  "Truster 7" <- TRUE ("Truster 6")
                }
              }
              n279 = Greater Or Equal?(x=w98, y=w135) -> (x >= y?=w150:bool)
              n280 = Less Or Equal?(x=w98, y=w134) -> (x <= y?=w149:bool)
              n281 = Or(x=w150, y=w149) -> (x .or. y?=w148:bool)
              n282 = case shown="True" w150 {
                frame False {
                }
                frame True {
                  "Truster1" <- TRUE ("Truster 6")
                  "Truster 6" <- TRUE ("Truster 6")
                  "Truster  2" <- FALSE ("Truster 6")
                  "Truster 5" <- FALSE ("Truster 6")
                }
              }
              n283 = case shown="False" w148 {
                frame False {
                  n284 = local write "Truster  2"(FALSE ("Truster 6")) -> ()
                  n285 = local write "Truster 6"(FALSE ("Truster 6")) -> ()
                  n286 = local write "Truster1"(FALSE ("Truster 6")) -> ()
                  n287 = local write "Truster 5"(FALSE ("Truster 6")) -> ()
                }
                frame True {
                }
              }
              n288 = case shown="True" w149 {
                frame False {
                }
                frame True {
                  n289 = local write "Truster  2"(TRUE ("Truster 6")) -> ()
                  n290 = local write "Truster 5"(TRUE ("Truster 6")) -> ()
                  n291 = local write "Truster1"(FALSE ("Truster 6")) -> ()
                  n292 = local write "Truster 6"(FALSE ("Truster 6")) -> ()
                }
              }
            }
          }
          n293 = local read "退出程序"() -> (w83:bool)
          n294 = node-c288() -> ()  [unwired: 1 in, 1 out]
        }
        n295 = call-poly <vilib>:"DAQmx Create Virtual Channel.vi"("lines"=tag "Dev1/port0/line7:15" ("Lines"), "line grouping"=w56) -> ("task out"=w61:refnum<k21>, "error out"=w60:errorcluster)  [unwired: 12 in]
        n296 = call <vilib>:"DAQmx Start Task.vi"("task/channels in"=w61, "error in"=w60) -> ("task out"=w63:refnum<k21>, "error out"=w66:errorcluster)  [unwired: 12 in]
        n297 = while {
          tunnel: w66 -> [w253]
          tunnel: [w254] -> w65
          tunnel: w63 -> [w256]
          tunnel: [w255] -> w62
          stop <- w257 stop-if-true
          n298 = Wait Until Next ms Multiple(millisecond multiple=u32 50) -> ()  [unwired: 1 out]
          n299 = local read "Truster  2"() -> (w250:bool)
          n300 = local read "Truster 5"() -> (w251:bool)
          n301 = local read "Truster1"() -> (w249:bool)
          n302 = local read "Truster 7"() -> (w243:bool)
          n303 = local read "Truster 6"() -> (w248:bool)
          n304 = local read "Truster4"() -> (w244:bool)
          n305 = local read "Truster 8"() -> (w245:bool)
          n306 = local read "Truster  3"() -> (w246:bool)
          n307 = call "Thruster8.vi"("Thruster 2"=w250, "Truster1"=w249, "Floating"="Floating", "Thruster 3"=w246, "Thruster 8"=w245, "task in"=w256, "Thruster 4"=w244, "Thruster 7"=w243, "Thruster 5"=w251, "error in"=w253, "Thruster 6"=w248) -> ("task out"=w255:refnum<k21>, "error out"=w254:errorcluster)  [unwired: 3 in]
          n308 = local read "退出程序"() -> (w257:bool)
        }
        n309 = call <vilib>:"DAQmx Clear Task.vi"("task in"=w62, "error in"=w65) -> ("error out"=w64:errorcluster)  [unwired: 13 in]
        n310 = call <vilib>:"Simple Error Handler.vi"("type of dialog (OK msg:1)"=w58, "error in (no error)"=w64) -> ()  [unwired: 3 in, 5 out]
        n311 = VISA Close(VISA resource name=w78, error in (no error)=w77) -> ()  [unwired: 1 out]
        n312 = node-c288(w53) -> ()  [unwired: 1 out]
        "电机已启动" <- FALSE
      }
    }
    n313 = local read "打开"() -> (w3:bool)
    n314 = And(x=w3, y="退出程序") -> (x .and. y?=w1:bool)
    n315 = case shown="False" w1 {
      frame False {
      }
      frame True {
        n316 = local write "打开"(FALSE ("打开")) -> ()
      }
    }
    "串口状态" <- "打开"
  }
